vi "FlipstogramDual.vi"(4 "intervals":i32=22, 6 "Array2":dbl[](array[numeric]), 8 "Array1":dbl[](array[numeric])) -> (1 "Flipst2":T1, 3 "Flipst1":T1)   [LabVIEW 2013]
doc: "Produces 2 histograms, sharing common bins"
uses:
  <vilib>/Analysis/NI_AALPro.lvlib
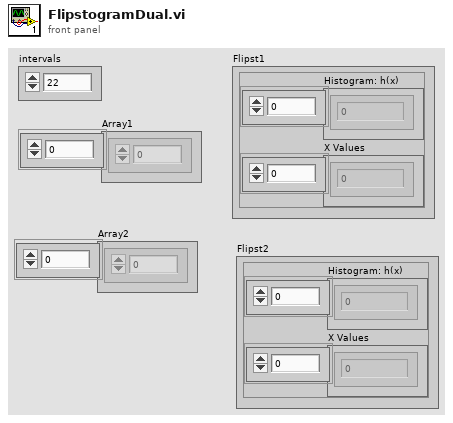
[diagram p1: front panel]
types:
  T1 = cluster{"Histogram: h(x)":i32[], "X Values":dbl[]}
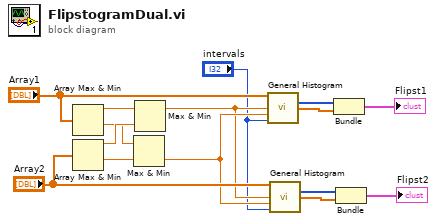
[diagram p0: block diagram]
diagram:
  n1 = Array Max & Min(array="Array1") -> (max value=w15:dbl, min value=w13:dbl)  [unwired: 2 out]
  n2 = Array Max & Min(array="Array2") -> (max value=w14:dbl, min value=w12:dbl)  [unwired: 2 out]
  n3 = Max & Min(x=w13, y=w12) -> (min(x,y)=w5:dbl)  [unwired: 1 out]
  n4 = Max & Min(x=w15, y=w14) -> (max(x,y)=w4:dbl)  [unwired: 1 out]
  n5 = call <vilib>:"General Histogram.vi"("X"="Array1", "max"=w4, "min"=w5, "# bins"="intervals") -> ("Histogram"=w11:i32[], "Axis"=w10:dbl[])  [unwired: 7 in, 3 out]
  n6 = call <vilib>:"General Histogram.vi"("X"="Array2", "max"=w4, "min"=w5, "# bins"="intervals") -> ("Histogram"=w7:i32[], "Axis"=w8:dbl[])  [unwired: 7 in, 3 out]
  n7 = Bundle("Histogram"=w11, "Axis"=w10) -> (→"Flipst1":cluster{"Histogram":i32[], "Axis":dbl[]})  [unwired: 1 in]
  n8 = Bundle("Histogram"=w7, "Axis"=w8) -> (→"Flipst2":cluster{"Histogram":i32[], "Axis":dbl[]})  [unwired: 1 in]
